vi "Untitled 2.vi"() -> ()   [LabVIEW 2018]
panel:
  in  "Numeric":dbl
  out "Boolean 7":bool
  out "Boolean 6":bool
  out "Boolean 5":bool
  out "Boolean 4":bool
  out "Boolean 3":bool
  out "Boolean 2":bool
  out "Boolean":bool
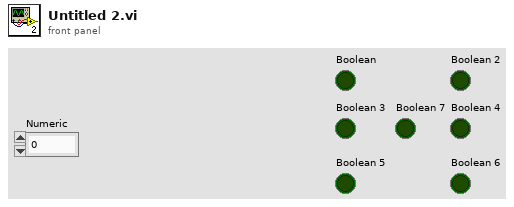
[diagram p1: front panel]
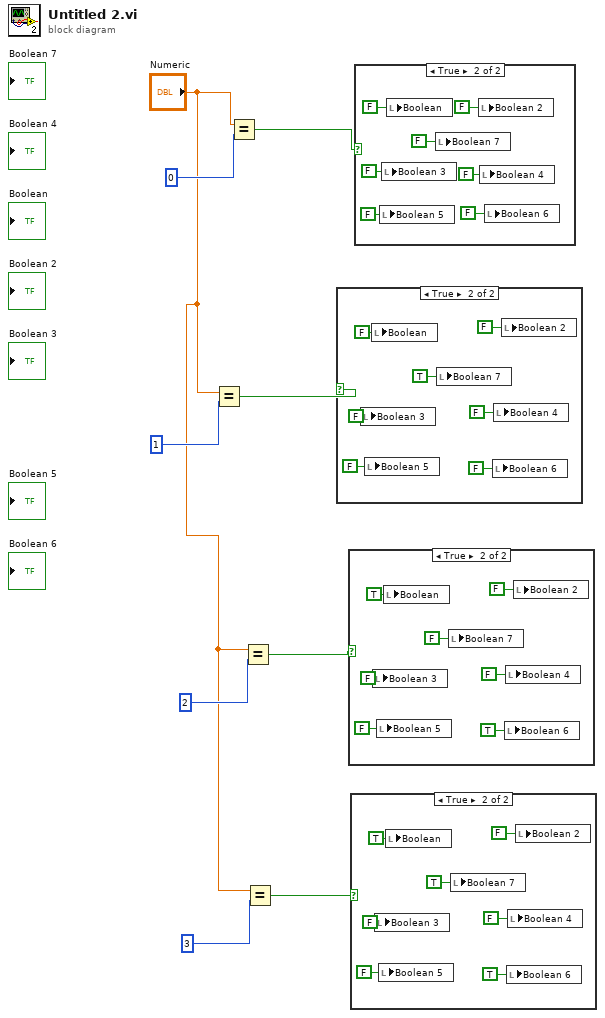
[diagram p0: block diagram]
diagram:
  n1 = Equal?(x="Numeric", y=1) -> (x = y?=w6:bool)
  n2 = Equal?(x="Numeric", y=0) -> (x = y?=w8:bool)
  n3 = Equal?(x="Numeric", y=2) -> (x = y?=w4:bool)
  n4 = Equal?(x="Numeric", y=3) -> (x = y?=w2:bool)
  n5 = case shown="True" w6 {
    frame False {
    }
    frame True {
      n6 = local write "Boolean 3"(FALSE ("Boolean 3")) -> ()
      n7 = local write "Boolean 5"(FALSE ("Boolean 5")) -> ()
      n8 = local write "Boolean"(FALSE ("Boolean")) -> ()
      n9 = local write "Boolean 7"(TRUE ("Boolean 7")) -> ()
      n10 = local write "Boolean 6"(FALSE ("Boolean 6")) -> ()
      n11 = local write "Boolean 4"(FALSE ("Boolean 4")) -> ()
      n12 = local write "Boolean 2"(FALSE ("Boolean 2")) -> ()
    }
  }
  n13 = case shown="True" w4 {
    frame False {
    }
    frame True {
      n14 = local write "Boolean 3"(FALSE ("Boolean 3")) -> ()
      n15 = local write "Boolean 5"(FALSE ("Boolean 5")) -> ()
      n16 = local write "Boolean"(TRUE ("Boolean")) -> ()
      n17 = local write "Boolean 7"(FALSE ("Boolean 7")) -> ()
      n18 = local write "Boolean 6"(TRUE ("Boolean 6")) -> ()
      n19 = local write "Boolean 4"(FALSE ("Boolean 4")) -> ()
      n20 = local write "Boolean 2"(FALSE ("Boolean 2")) -> ()
    }
  }
  n21 = case shown="True" w2 {
    frame False {
    }
    frame True {
      n22 = local write "Boolean 3"(FALSE ("Boolean 3")) -> ()
      n23 = local write "Boolean 5"(FALSE ("Boolean 5")) -> ()
      n24 = local write "Boolean"(TRUE ("Boolean")) -> ()
      n25 = local write "Boolean 7"(TRUE ("Boolean 7")) -> ()
      n26 = local write "Boolean 6"(TRUE ("Boolean 6")) -> ()
      n27 = local write "Boolean 4"(FALSE ("Boolean 4")) -> ()
      n28 = local write "Boolean 2"(FALSE ("Boolean 2")) -> ()
    }
  }
  n29 = case shown="True" w8 {
    frame False {
    }
    frame True {
      n30 = local write "Boolean 5"(FALSE ("Boolean 5")) -> ()
      n31 = local write "Boolean 3"(FALSE ("Boolean 3")) -> ()
      n32 = local write "Boolean"(FALSE ("Boolean")) -> ()
      n33 = local write "Boolean 7"(FALSE ("Boolean 7")) -> ()
      n34 = local write "Boolean 2"(FALSE ("Boolean 2")) -> ()
      n35 = local write "Boolean 4"(FALSE ("Boolean 4")) -> ()
      n36 = local write "Boolean 6"(FALSE ("Boolean 6")) -> ()
    }
  }
